vi "CRYSelect New Name.vi"(4 "Result":T1, 6 "Type":string, 7 "Option":string, 8 "Wave":T1, 9 "Value":T1, 10 "Curve":T1, 11 "Name In":string) -> (0 "Change":bool, 1 "Status":string, 3 "Name Out":string)   [LabVIEW 2013]
uses:
  CRYSystem/Typedef Control/CRYChanged Data Array Cluster.ctl
  CRYSystem/Typedef Control/CRYChanged Data Cluster.ctl
panel:
  in  "Temp":string
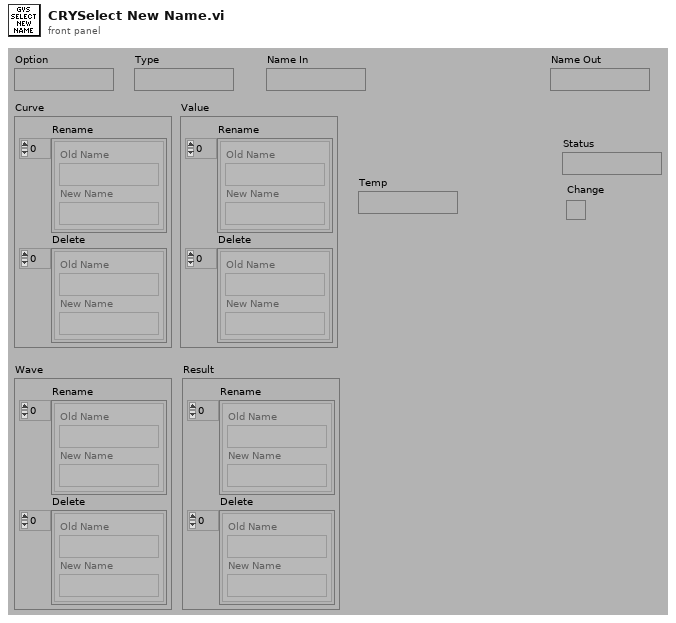
[diagram p1: front panel]
types:
  T1 = typedef "CRYChanged Data Array Cluster.ctl" = cluster{"Rename":T2[], "Delete":T2[]}
  T2 = typedef "CRYChanged Data Cluster.ctl" = cluster{"Old Name":string, "New Name":string}
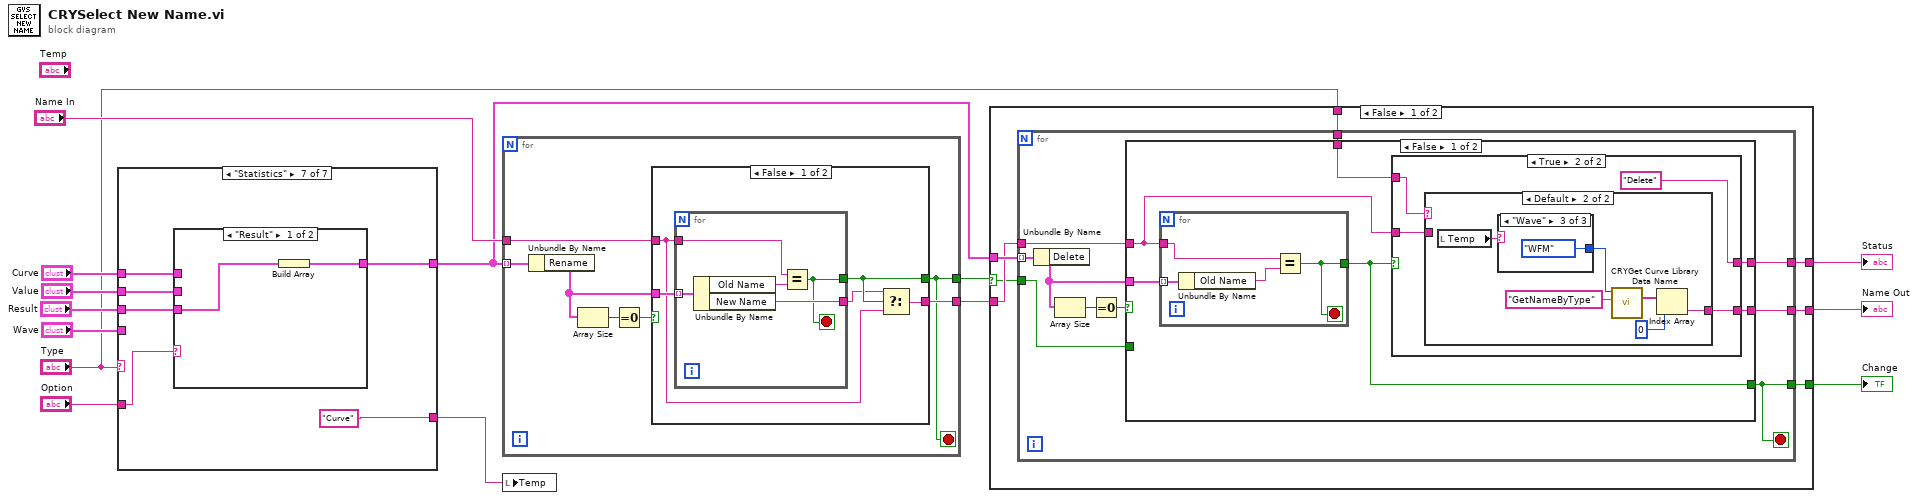
[diagram p0: block diagram]
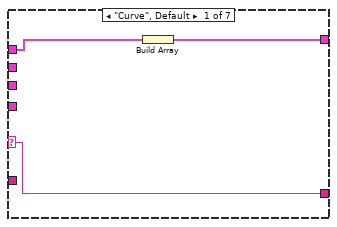
[diagram p2: hidden frame]
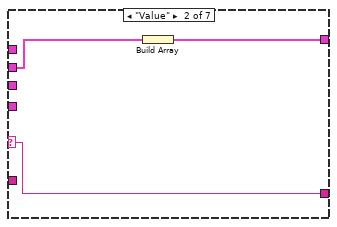
[diagram p3: hidden frame]
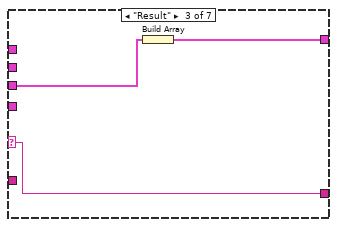
[diagram p4: hidden frame]
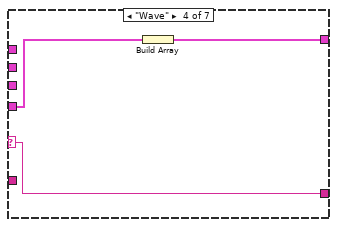
[diagram p5: hidden frame]
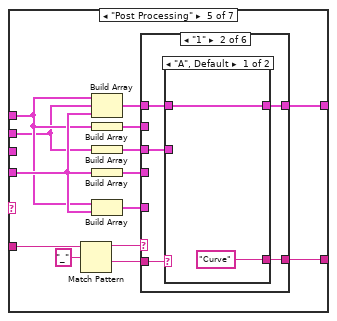
[diagram p6: hidden frame]
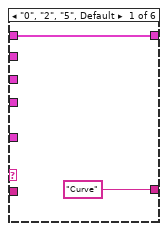
[diagram p7: hidden frame]
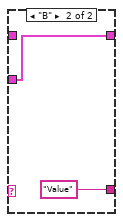
[diagram p8: hidden frame]
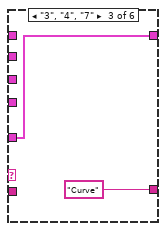
[diagram p9: hidden frame]
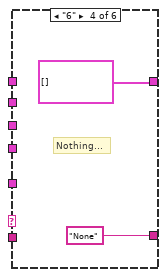
[diagram p10: hidden frame]
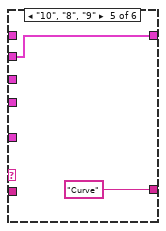
[diagram p11: hidden frame]
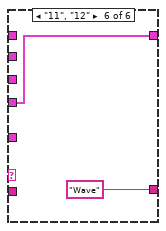
[diagram p12: hidden frame]
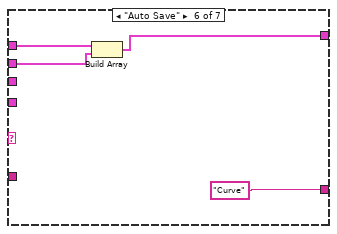
[diagram p13: hidden frame]
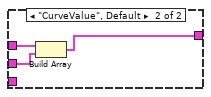
[diagram p14: hidden frame]
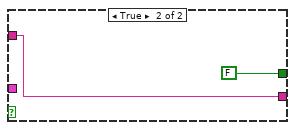
[diagram p15: hidden frame]
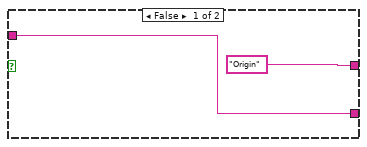
[diagram p16: hidden frame]
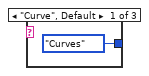
[diagram p18: hidden frame]
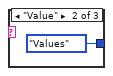
[diagram p19: hidden frame]
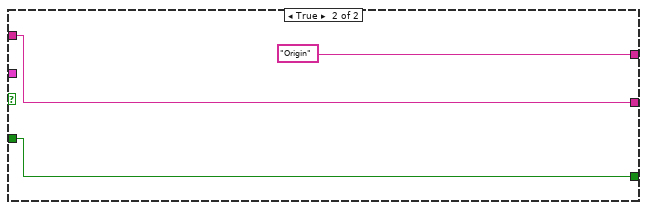
[diagram p20: hidden frame]
diagram:
  n1 = case shown="\"Statistics\"" "Type" {
    selector: "Type" -> [w15 w18 w21 w24 _ _ _]
    tunnel: "Wave" -> [_ _ _ w25 w40 _ _]
    tunnel: "Curve" -> [w17 _ _ _ w39 w63 w69]
    tunnel: "Value" -> [_ w19 _ _ w38 w61 w67]
    tunnel: "Option" -> [_ _ _ _ w32 _ w65]
    tunnel: [w15 w18 w21 w24 w28 "Curve" ("Temp") "Curve" ("Temp")] -> w5
    tunnel: [w16 w20 w23 w26 w27 w60 w66] -> w4
    tunnel: "Result" -> [_ _ w22 _ _ _ w64]
    frame "Curve", Default {
      n2 = Build Array(w17) -> (w16:T1[])
    }
    frame "Value" {
      n3 = Build Array(w19) -> (w20:T1[])
    }
    frame "Result" {
      n4 = Build Array(w22) -> (w23:T1[])
    }
    frame "Wave" {
      n5 = Build Array(w25) -> (w26:T1[])
    }
    frame "Post Processing" {
      n6 = Match Pattern(string=w32, regular expression="_") -> (before substring=w30:string, after substring=w29:string)  [unwired: 1 in, 2 out]
      n7 = Build Array(w39, w38, w40) -> (w37:T1[])
      n8 = Build Array(w39) -> (w36:T1[])
      n9 = Build Array(w38) -> (w35:T1[])
      n10 = Build Array(w40) -> (w34:T1[])
      n11 = Build Array(w39, w40) -> (w33:T1[])
      n12 = case shown="\"1\"" w30 {
        tunnel: w37 -> [w42 w44 _ _ _ _]
        tunnel: w36 -> [_ _ _ _ w56 _]
        tunnel: w35 -> [_ w43 _ _ _ _]
        tunnel: w34 -> [_ _ _ _ _ w58]
        tunnel: w33 -> [_ _ w53 _ _ _]
        tunnel: [w42 w46 w53 T1[] [] ("appended array") w56 w58] -> w27
        tunnel: w29 -> [_ w47 _ _ _ _]
        tunnel: ["Curve" ("Temp") w45 "Curve" ("Temp") "None" ("Temp") "Curve" ("Temp") "Wave" ("Temp")] -> w28
        frame "0", "2", "5", Default {
        }
        frame "1" {
          n13 = case shown="\"A\", Default" w47 {
            tunnel: w44 -> [w49 _]
            tunnel: [w49 w50] -> w46
            tunnel: ["Curve" ("Temp") "Value" ("Temp")] -> w45
            tunnel: w43 -> [_ w50]
            frame "A", Default {
            }
            frame "B" {
            }
          }
        }
        frame "3", "4", "7" {
        }
        frame "6" {
          # "Nothing..."
        }
        frame "10", "8", "9" {
        }
        frame "11", "12" {
        }
      }
    }
    frame "Auto Save" {
      n14 = Build Array(w63, w61) -> (w60:T1[])
    }
    frame "Statistics" {
      n15 = case shown="\"Result\"" w65 {
        tunnel: w69 -> [_ w74]
        tunnel: w67 -> [_ w73]
        tunnel: [w70 w72] -> w66
        tunnel: w64 -> [w71 _]
        frame "Result" {
          n16 = Build Array(w71) -> (w70:T1[])
        }
        frame "CurveValue", Default {
          n17 = Build Array(w74, w73) -> (w72:T1[])
        }
      }
    }
  }
  n18 = for {
    tunnel: "Name In" -> [w81]
    tunnel: [w77] -> w7
    tunnel: [w76] -> w6
    tunnel: w4 -> [w75] mode=indexing
    stop <- w76 stop-if-true
    n19 = Unbundle By Name(w75) -> ("Rename"=w79:T2[])
    n20 = Array Size(array=w79) -> (size(s)=w80:i32)
    n21 = Equal To 0?(x=w80) -> (x = 0?=w78:bool)
    n22 = case shown="False" w78 {
      tunnel: w79 -> [w86 _]
      tunnel: w81 -> [w83 w92]
      tunnel: [w82 w92] -> w77
      tunnel: [w85 FALSE] -> w76
      frame False {
        n23 = for {
          tunnel: w86 -> [w91] mode=indexing
          tunnel: w83 -> [w89]
          tunnel: [w88] -> w84
          tunnel: [w87] -> w85
          stop <- w87 stop-if-true
          n24 = Unbundle By Name(w91) -> ("Old Name"=w90:string, "New Name"=w88:string)
          n25 = Equal?(x=w89, y=w90) -> (x = y?=w87:bool)
        }
        n26 = Select(t=w84, s=w85, f=w83) -> (s? t:f=w82:string)
      }
      frame True {
      }
    }
  }
  n27 = local write "Temp"(w5) -> ()
  n28 = case shown="False" w6 {
    selector: w6 -> [w97 w141]
    tunnel: [w98 w142] -> w12
    tunnel: w7 -> [w99 w142]
    tunnel: w4 -> [w100 _]
    tunnel: [w96 w141] -> w3
    tunnel: "Type" -> [w95 _]
    tunnel: [w94 "Rename" ("Status")] -> w1
    frame False {
      n29 = for {
        tunnel: w100 -> [w107] mode=indexing
        tunnel: w99 -> [w106]
        tunnel: [w105] -> w98
        tunnel: w97 -> [w104]
        tunnel: [w103] -> w96
        tunnel: w95 -> [w102]
        tunnel: [w101] -> w94
        stop <- w103 stop-if-true
        n30 = Unbundle By Name(w107) -> ("Delete"=w110:T2[])
        n31 = Array Size(array=w110) -> (size(s)=w108:i32)
        n32 = Equal To 0?(x=w108) -> (x = 0?=w109:bool)
        n33 = case shown="False" w109 {
          tunnel: w110 -> [w116 _]
          tunnel: w106 -> [w114 w139]
          tunnel: [w115 w139] -> w105
          tunnel: w104 -> [_ w138]
          tunnel: [w113 w138] -> w103
          tunnel: w102 -> [w112 _]
          tunnel: [w111 "Origin"] -> w101
          frame False {
            n34 = for {
              tunnel: w114 -> [w135]
              tunnel: w116 -> [w136] mode=indexing
              tunnel: [w133] -> w113
              stop <- w133 stop-if-true
              n35 = Unbundle By Name(w136) -> ("Old Name"=w134:string)
              n36 = Equal?(x=w135, y=w134) -> (x = y?=w133:bool)
            }
            n37 = case shown="True" w113 {
              tunnel: [w118 w122] -> w115
              tunnel: w114 -> [w118 w119]
              tunnel: w112 -> [_ w121]
              tunnel: ["Origin" "Delete" ("Status")] -> w111
              frame False {
              }
              frame True {
                n38 = case shown="Default" w121 {
                  tunnel: [w123 w126] -> w122
                  tunnel: w119 -> [w123 _]
                  frame "Statistics" {
                  }
                  frame Default {
                    n39 = local read "Temp"() -> (w125:string)
                    n40 = case shown="\"Wave\"" w125 {
                      tunnel: [enum16{"Curves", "Values", "Results", "WFM"}."Curves" ("Type") enum16{"Curves", "Values", "Results", "WFM"}."Values" ("Type") enum16{"Curves", "Values", "Results", "WFM"}."WFM" ("Type")] -> w124
                      frame "Curve", Default {
                      }
                      frame "Value" {
                      }
                      frame "Wave" {
                      }
                    }
                    n41 = call "CRYGet Curve Library Data Name.vi"("sAction"="GetNameByType", "Type"=w124) -> ("sNames"=w128:string[])  [unwired: 6 in, 3 out]
                    n42 = Index Array(array=w128, index=0) -> (element=w126:string)
                  }
                }
              }
            }
          }
          frame True {
          }
        }
      }
    }
    frame True {
    }
  }
  "Name Out" <- w12
  "Change" <- w3
  "Status" <- w1
